vi "validate.vi"(8 "error in":errorcluster, 11 "io configuration in":refnum<class "io configuration.lvclass">) -> (0 "error out":errorcluster, 3 "io configuration out":refnum<class "io configuration.lvclass">)   [LabVIEW 2015, in "io configuration.lvclass"]
doc: "This function performs validation of the configuration. This function should be safe to call at any point and should not rely on anything in the runtime environment."
uses:
  io configuration.lvclass
  io configuration.lvclass/io configuration.ctl
  Read Resource.vi
  Read Bitfile path.vi
  Read Bitfile exe dir.vi
  Read Load FPGA.vi
  <vilib>/NI/Tag Bus Module Framework/module configuration/TBM module configuration.lvclass
  <vilib>/NI/Configuration Framework/NISE_CEF_TreeControl.lvlib
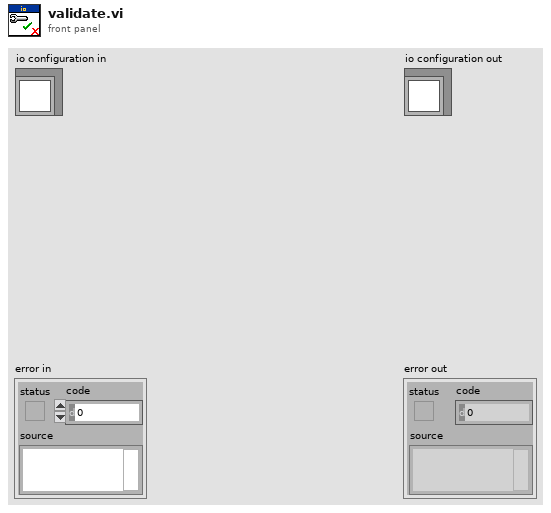
[diagram p1: front panel]
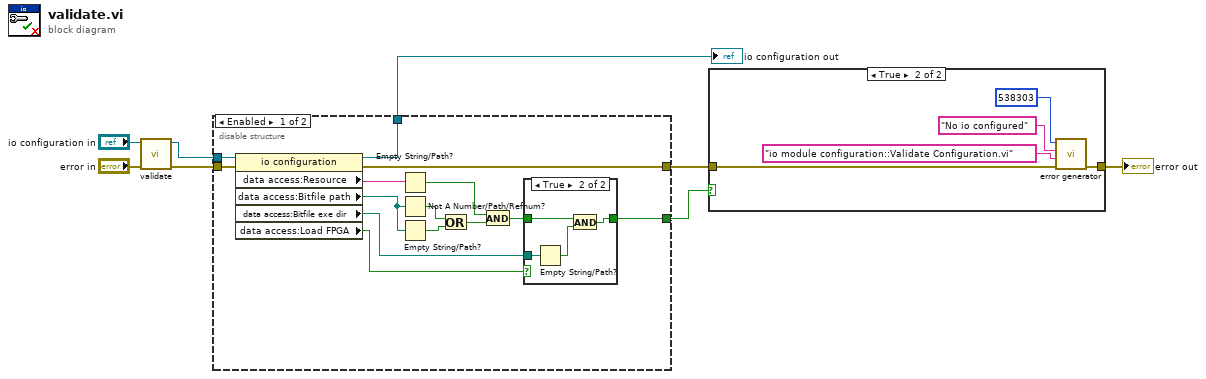
[diagram p0: block diagram]
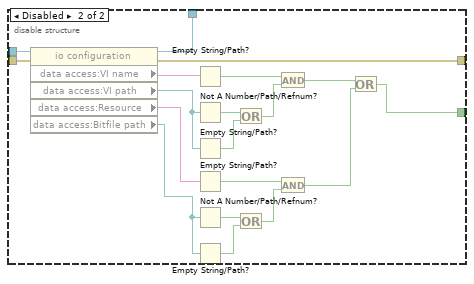
[diagram p3: hidden frame]
diagram:
  n1 = call-parent "validate.vi"("error in"="error in", "configuration in"="io configuration in") -> ("error out"=w8:errorcluster, "configuration out"=w5:refnum<class "io configuration.lvclass">)  [unwired: 8 in]
  n2 = disable-structure shown="Enabled" {
    disable-tunnel: w8 -> [w22 w46]
    disable-tunnel: w5 -> [w21 w45]
    disable-tunnel: [w20 w44] -> w4
    disable-tunnel: [w19 w43] -> w3
    disable-tunnel: [w9 w30] -> w1
    frame Enabled {
      n3 = property class="io configuration"(reference=w21, error in=w22) -> (reference out=w20:refnum<class "io configuration.lvclass">, error out=w19:errorcluster, "data access:Resource"=w18:string, "data access:Bitfile path"=w13:path, "data access:Bitfile exe dir"=w11:path, "data access:Load FPGA"=w12:bool)
      n4 = Empty String/Path?(string/path=w18) -> (empty?=w17:bool)
      n5 = Not A Number/Path/Refnum?(number/path/refnum=w13) -> (NaN/Path/Refnum?=w15:bool)
      n6 = Empty String/Path?(string/path=w13) -> (empty?=w16:bool)
      n7 = Or(x=w15, y=w16) -> (x .or. y?=w14:bool)
      n8 = And(x=w17, y=w14) -> (x .and. y?=w10:bool)
      n9 = case shown="True" w12 {
        tunnel: w11 -> [_ w27]
        tunnel: w10 -> [w23 w26]
        tunnel: [w23 w24] -> w9
        frame False {
        }
        frame True {
          n10 = Empty String/Path?(string/path=w27) -> (empty?=w25:bool)
          n11 = And(x=w26, y=w25) -> (x .and. y?=w24:bool)
        }
      }
    }
    frame Disabled {
      n12 = property class="io configuration"(reference=w45, error in=w46) -> (reference out=w44:refnum<class "io configuration.lvclass">, error out=w43:errorcluster, "data access:VI name"=w42:string, "data access:VI path"=w37:path, "data access:Resource"=w32:string, "data access:Bitfile path"=w31:path)
      n13 = Empty String/Path?(string/path=w42) -> (empty?=w41:bool)
      n14 = Not A Number/Path/Refnum?(number/path/refnum=w37) -> (NaN/Path/Refnum?=w39:bool)
      n15 = Empty String/Path?(string/path=w37) -> (empty?=w40:bool)
      n16 = Empty String/Path?(string/path=w32) -> (empty?=w33:bool)
      n17 = Not A Number/Path/Refnum?(number/path/refnum=w31) -> (NaN/Path/Refnum?=w35:bool)
      n18 = Empty String/Path?(string/path=w31) -> (empty?=w34:bool)
      n19 = Or(x=w39, y=w40) -> (x .or. y?=w38:bool)
      n20 = Or(x=w35, y=w34) -> (x .or. y?=w36:bool)
      n21 = And(x=w41, y=w38) -> (x .and. y?=w29:bool)
      n22 = And(x=w33, y=w36) -> (x .and. y?=w28:bool)
      n23 = Or(x=w29, y=w28) -> (x .or. y?=w30:bool)
    }
  }
  "io configuration out" <- w4
  n24 = case shown="True" w1 {
    tunnel: w3 -> [w47 w49]
    tunnel: [w47 w48] -> w2
    frame False {
    }
    frame True {
      n25 = call <vilib>:"error generator.vi"("error in"=w49, "source"="io module configuration::Validate Configuration.vi", "append error message"="No io configured", "error code (0)"=538303) -> ("error out"=w48:errorcluster)  [unwired: 5 in]
    }
  }
  "error out" <- w2
